vi "qFRC.vi"(0 "System no.":i32=1 min=1 max=4 step=1, 2 "Routines to query":string[](array[string]), 3 "All routines?":bool, 5 "error in":errorcluster) -> (14 "Routines coupled":string[][](array[string]), 19 "error out":errorcluster)   [LabVIEW 2026]
doc: "Returns fast alignment routine coupling.\n\nC-887, E-712:"
panel:
  # "Query Fast alignment Routine Coupling"
  # "Query"
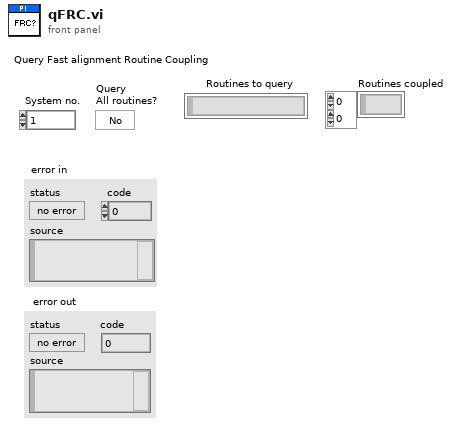
[diagram p1: front panel]
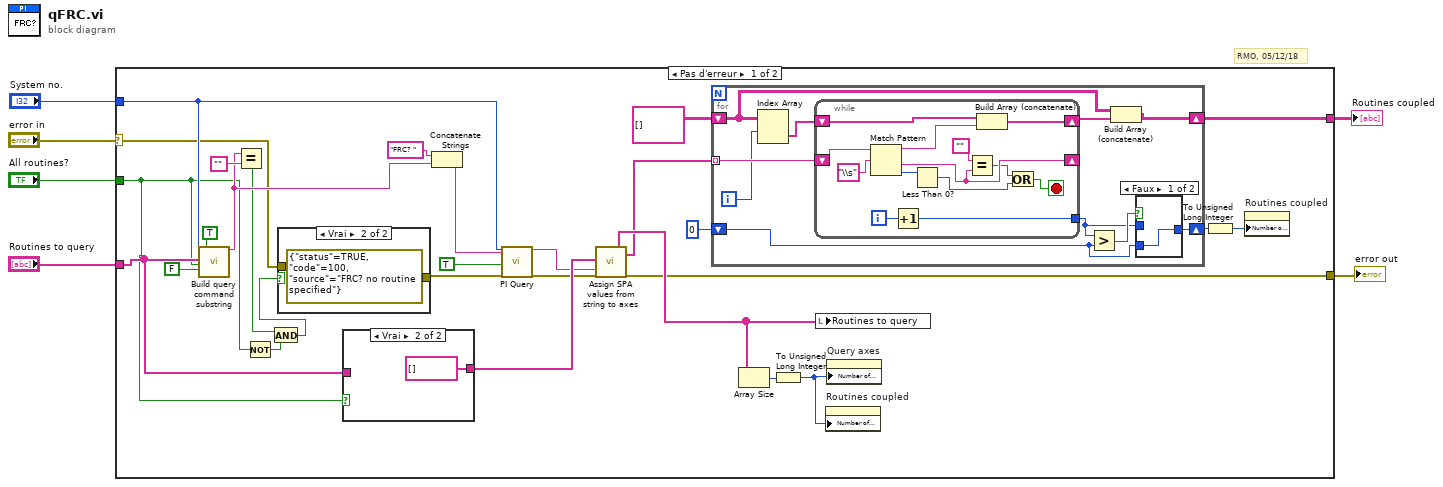
[diagram p0: block diagram]
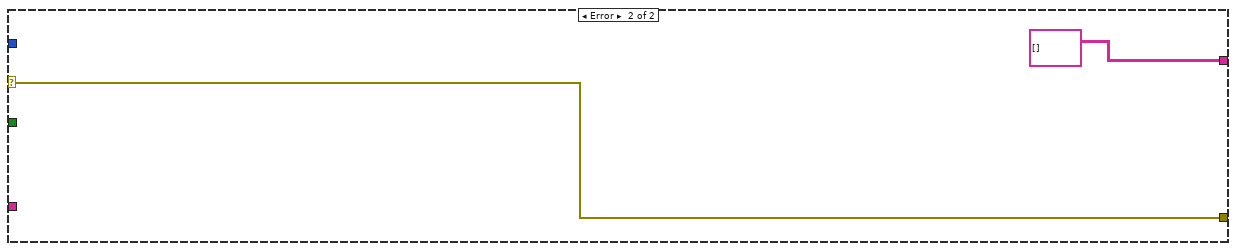
[diagram p5: hidden frame]
diagram:
  # "RMO, 05/12/18"
  n1 = case shown="Pas d'erreur" "error in" {
    selector: "error in" -> [w9 w64]
    tunnel: "Routines to query" -> [w12 _]
    tunnel: [w19 w64] -> w5
    tunnel: "System no." -> [w20 _]
    tunnel: "All routines?" -> [w10 _]
    tunnel: [w21 string[][] []] -> w2
    frame No Error {
      n2 = call "Build query command substring.vi"("System no."=w20, "Axes to query in"=w12, "Query\nAll axes?"=w10, "For all axes: use\nAxis identifier?"=FALSE ("For all axes: use\nAxis identifier?"), "With space?"=TRUE) -> ("Command substring"=w29:string)  [unwired: 1 in, 13 out]
      n3 = Equal?(x=w29, y="" ("x")) -> (x = y?=w28:bool)
      n4 = Not(x=w10) -> (.not. x?=w27:bool)
      n5 = And(x=w28, y=w27) -> (x .and. y?=w30:bool)
      n6 = case shown="Vrai" w30 {
        tunnel: [w62 errorcluster {"status"=TRUE, "code"=100, "source"="FRC? no routine specified"} ("error out")] -> w24
        tunnel: w9 -> [w62 _]
        frame False {
        }
        frame True {
        }
      }
      n7 = case shown="Vrai" w10 {
        tunnel: w12 -> [w35 _]
        tunnel: [w35 string[] [] ("Routines to query")] -> w11
        frame False {
        }
        frame True {
        }
      }
      n8 = Concatenate Strings("FRC? ", w29) -> (w32:string)
      n9 = call "PI Query.vi"("System no."=w20, "String to send"=w32, "Attach termination char.?"=TRUE ("Attach Linefeed?"), "error in"=w24) -> ("String read"=w7:string, "error out"=w8:errorcluster)  [unwired: 3 in, 11 out]
      n10 = call "Assign SPA values from string to axes.vi"("Queried axes"=w11, "Input string"=w7, "error in"=w8) -> ("Queried axes out"=w23:string[], "Parameter strings"=w18:string[], "error out"=w19:errorcluster)  [unwired: 4 in, 10 out]
      n11 = for {
        tunnel: w18 -> [w46] mode=indexing
        shift-right: [w45] -> w21
        shift-left: string[][] [] -> [w43]
        shift-right: [w38] -> w13
        shift-left: 0 -> [w37]
        i -> [w42]
        n12 = Index Array(array=w43, index (row)=w42) -> (element=w41:string[])  [unwired: 1 in]
        n13 = while {
          shift-right: [w57] -> w44
          shift-left: w41 -> [w59]
          shift-right: [w55] -> _
          shift-left: w46 -> [w61]
          tunnel: [w49] -> w39
          i -> [w50]
          stop <- w52 stop-if-true
          n14 = Match Pattern(string=w61, regular expression="\\s") -> (before substring=w58:string, after substring=w55:string, offset past match=w56:i32)  [unwired: 2 out]
          n15 = Increment(x=w50) -> (x+1=w49:i32)
          n16 = Less Than 0?(x=w56) -> (x < 0?=w53:bool)
          n17 = Equal?(x="", y=w55) -> (x = y?=w51:bool)
          n18 = Build Array (concatenate)(w59, w58) -> (w57:string[])
          n19 = Or(x=w51, y=w53) -> (x .or. y?=w52:bool)
        }
        n20 = Greater?(x=w39, y=w37) -> (0:w40:bool)
        n21 = Build Array (concatenate)(w43, w44) -> (w45:string[][])
        n22 = case shown="Faux" w40 {
          tunnel: w39 -> [_ w48]
          tunnel: [w47 w48] -> w38
          tunnel: w37 -> [w47 _]
          frame False {
          }
          frame True {
          }
        }
      }
      n23 = Array Size(array=w23) -> (size(s)=w17:i32)
      n24 = To Unsigned Long Integer(number=w17) -> (unsigned 32bit integer=w16:u32)
      n25 = local write "Routines to query"(w23) -> ()
      n26 = property on="Routines coupled" class="Tabl (strict)"("Number of Rows"=w16) -> ()  [unwired: 2 in, 2 out]
      n27 = property on="Query axes" class="Tabl (strict)"("Number of Rows"=w16) -> ()  [unwired: 2 in, 2 out]
      n28 = To Unsigned Long Integer(number=w13) -> (unsigned 32bit integer=w14:u32)
      n29 = property on="Routines coupled" class="Tabl (strict)"("Number of Columns"=w14) -> ()  [unwired: 2 in, 2 out]
    }
    frame Error {
    }
  }
  "error out" <- w5
  "Routines coupled" <- w2
